vi "Get 2182 reading from 6221.vi"(0 "622x Resource In":refnum<visa-resource-name>, 1 "Check For SCPI Errors? (T)":bool=TRUE, 11 "error in (no error)":errorcluster) -> (4 "622x Resource Out (dupl)":refnum<visa-resource-name>, 6 "reading":dbl, 15 "error out":errorcluster)   [LabVIEW 2019, in "User lib.lvlib"]
uses:
  User lib.lvlib
  lib/Keithley 622x/Keithley 622x.lvlib
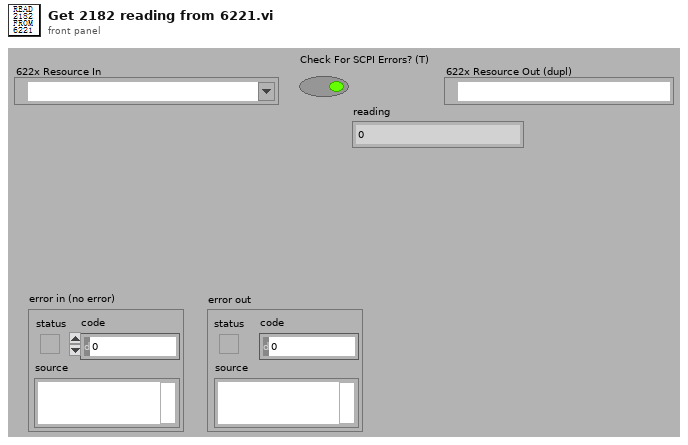
[diagram p1: front panel]
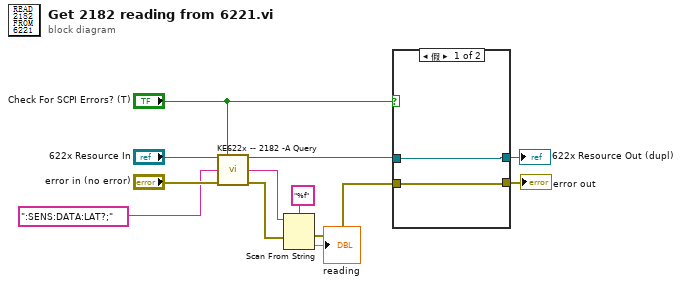
[diagram p0: block diagram]
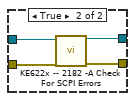
[diagram p2: hidden frame]
diagram:
  n1 = call "KE622x -- 2182 -A Query.vi"("622x Resource In"="622x Resource In", "Check For SCPI Errors? (T)"="Check For SCPI Errors? (T)", "2182-A Write String"=":SENS:DATA:LAT?;", "error in (no error)"="error in (no error)") -> ("622x Resource Out (dupl)"=w6:refnum<visa-resource-name>, "2182-A Reponse String"=w7:string, "error out"=w9:errorcluster)  [unwired: 9 in]
  n2 = Scan From String(format string="%f", input string=w7, error in=w9) -> (error out=w5:errorcluster, output 1=→"reading":dbl)  [unwired: 2 in, 2 out]
  n3 = case shown="假" "Check For SCPI Errors? (T)" {
    tunnel: w6 -> [w14 w18]
    tunnel: w5 -> [w13 w17]
    tunnel: [w14 w16] -> w3
    tunnel: [w13 w15] -> w2
    frame False {
    }
    frame True {
      n4 = call "KE622x -- 2182 -A Check For SCPI Errors.vi"("VISA Resource In"=w18, "error in (no error)"=w17) -> ("VISA Resource Out (dupl)"=w16:refnum<visa-resource-name>, "error out"=w15:errorcluster)  [unwired: 10 in, 2 out]
    }
  }
  "622x Resource Out (dupl)" <- w3
  "error out" <- w2
